vi "monte.fsk.vi"() -> ()   [LabVIEW 2014]
uses:
  <vilib>/Analysis/NI_AALBase.lvlib
panel:
  out "Waveform Chart":dbl(graph)
  in  "Numeric 4":i32
  in  "Numeric 2":i32
  out "BER":dbl format="%#_13g"
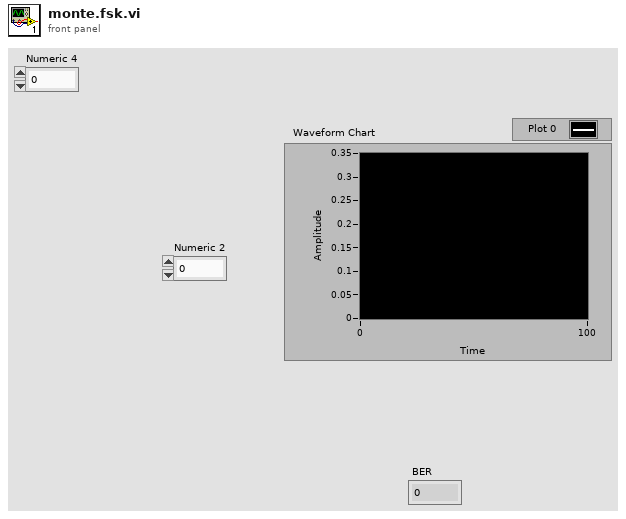
[diagram p1: front panel]
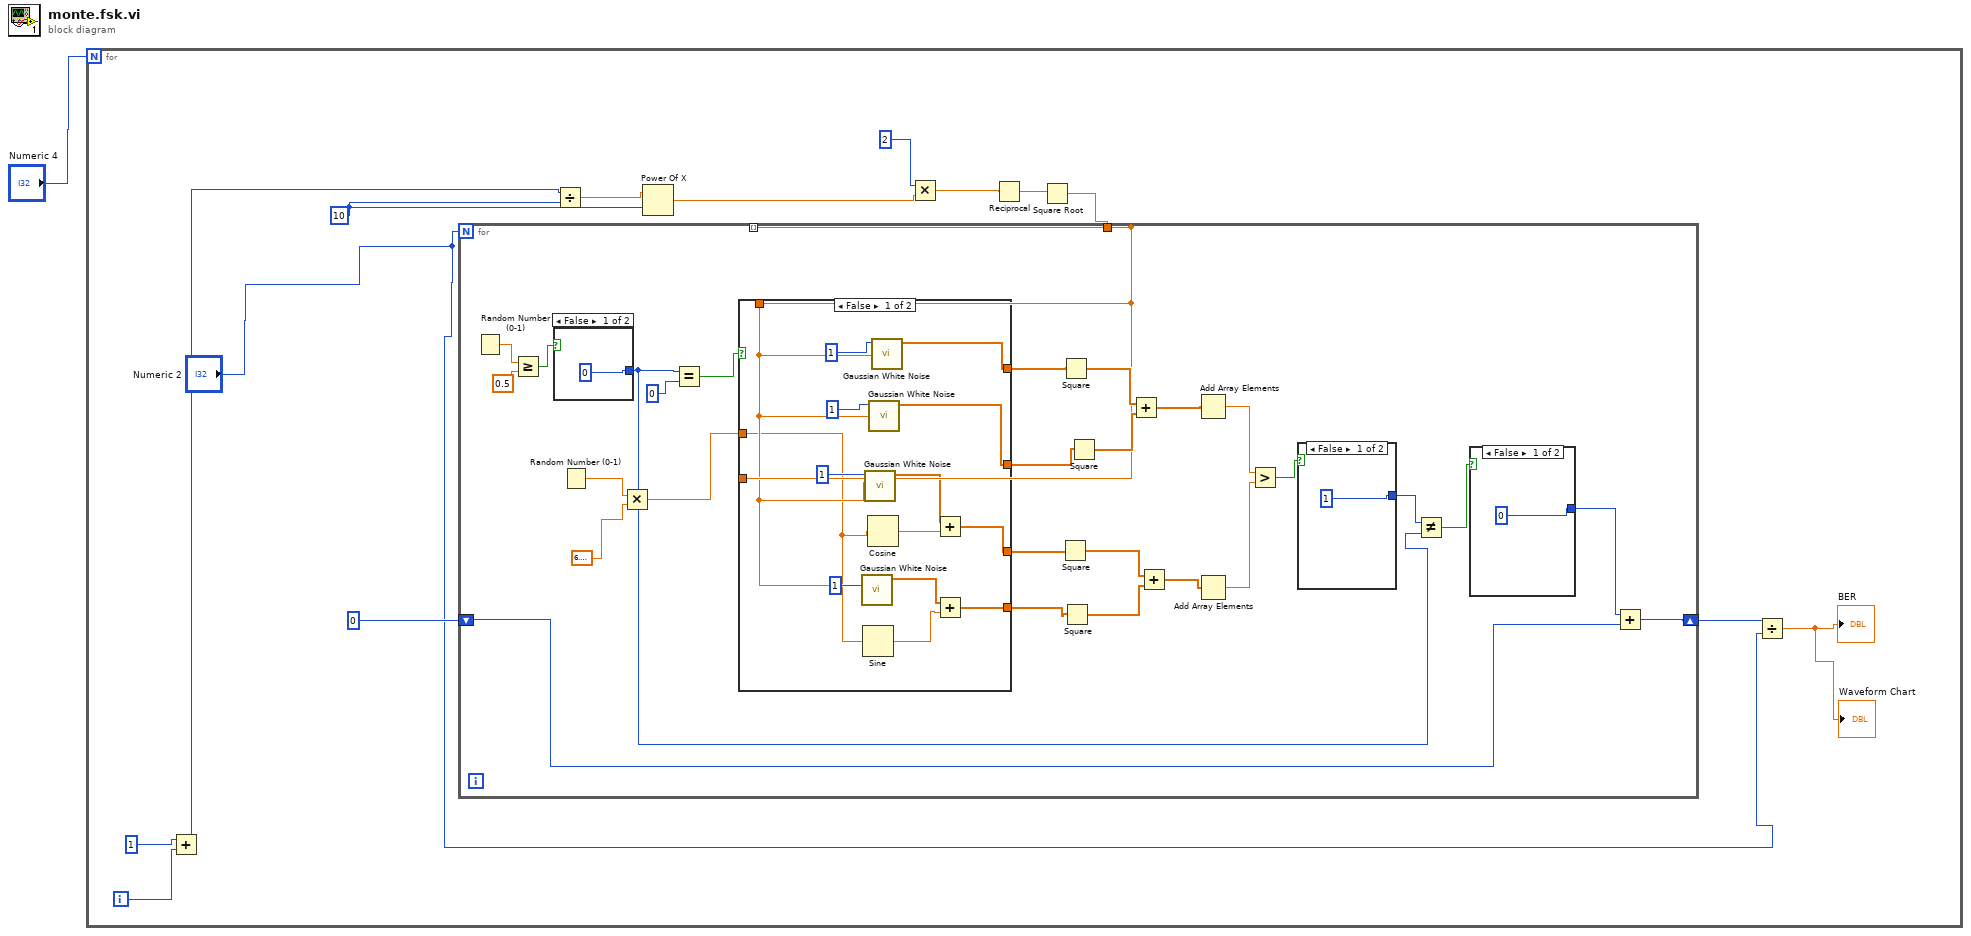
[diagram p0: block diagram]
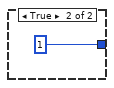
[diagram p2: hidden frame]
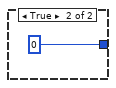
[diagram p3: hidden frame]
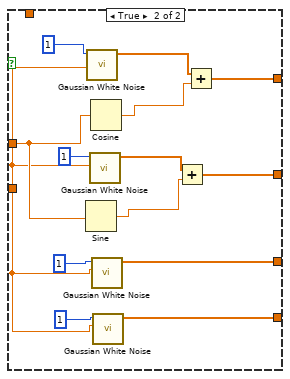
[diagram p4: hidden frame]
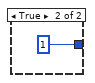
[diagram p5: hidden frame]
diagram:
  n1 = for {
    N: "Numeric 4" -> [_]
    i -> [w5]
    w13 = 10
    n2 = Add(x=1, y=w5) -> (x+y=w3:i32)
    n3 = Divide(x=w3, y=w13) -> (x/y=w14:dbl)
    n4 = Power Of X(1:w13, 2:w14) -> (0:w12:dbl)
    n5 = Multiply(x=2, y=w12) -> (x*y=w11:dbl)
    n6 = Reciprocal(x=w11) -> (1/x=w10:dbl)
    n7 = Square Root(x=w10) -> (sqrt(x)=w9:dbl)
    n8 = for {
      N: "Numeric 2" -> [_]
      shift-right: [w19] -> w15
      shift-left: 0 -> [w18]
      tunnel: [w16] -> _ mode=indexing
      tunnel: w9 -> [w16]
      n9 = Random Number (0-1)() -> (number: 0 to 1=w42:dbl)
      n10 = Greater Or Equal?(x=w42, y=0.5) -> (x >= y?=w43:bool)
      n11 = case shown="False" w43 {
        tunnel: [0 1] -> w21
        frame False {
        }
        frame True {
        }
      }
      n12 = Random Number (0-1)() -> (number: 0 to 1=w38:dbl)
      n13 = Multiply(x=w38, y=6.283185307179586) -> (x*y=w37:dbl)
      n14 = Equal?(x=w21, y=0) -> (x = y?=w39:bool)
      n15 = case shown="False" w39 {
        tunnel: w37 -> [w48 w63]
        tunnel: [w51 w74] -> w36
        tunnel: [w52 w71] -> w35
        tunnel: [w53 w70] -> w34
        tunnel: [w56 w69] -> w33
        tunnel: w16 -> [_ w62]
        tunnel: w16 -> [w49 _]
        frame False {
          n16 = call <vilib>:"Gaussian White Noise.vi"("standard deviation"=w49, "samples"=1) -> ("Gaussian noise pattern"=w58:dbl[])  [unwired: 8 in, 1 out]
          n17 = Sine(x=w48) -> (sin(x)=w57:dbl)
          n18 = call <vilib>:"Gaussian White Noise.vi"("standard deviation"=w49, "samples"=1) -> ("Gaussian noise pattern"=w54:dbl[])  [unwired: 8 in, 1 out]
          n19 = Cosine(x=w48) -> (cos(x)=w55:dbl)
          n20 = call <vilib>:"Gaussian White Noise.vi"("standard deviation"=w49, "samples"=1) -> ("Gaussian noise pattern"=w52:dbl[])  [unwired: 8 in, 1 out]
          n21 = call <vilib>:"Gaussian White Noise.vi"("standard deviation"=w49, "samples"=1) -> ("Gaussian noise pattern"=w51:dbl[])  [unwired: 8 in, 1 out]
          n22 = Add(x=w54, y=w55) -> (x+y=w53:dbl[])
          n23 = Add(x=w58, y=w57) -> (x+y=w56:dbl[])
        }
        frame True {
          n24 = Sine(x=w63) -> (sin(x)=w64:dbl)
          n25 = call <vilib>:"Gaussian White Noise.vi"("standard deviation"=w62, "samples"=1) -> ("Gaussian noise pattern"=w75:dbl[])  [unwired: 8 in, 1 out]
          n26 = call <vilib>:"Gaussian White Noise.vi"("standard deviation"=w62, "samples"=1) -> ("Gaussian noise pattern"=w72:dbl[])  [unwired: 8 in, 1 out]
          n27 = Cosine(x=w63) -> (cos(x)=w65:dbl)
          n28 = call <vilib>:"Gaussian White Noise.vi"("standard deviation"=w62, "samples"=1) -> ("Gaussian noise pattern"=w70:dbl[])  [unwired: 8 in, 1 out]
          n29 = call <vilib>:"Gaussian White Noise.vi"("standard deviation"=w62, "samples"=1) -> ("Gaussian noise pattern"=w69:dbl[])  [unwired: 8 in, 1 out]
          n30 = Add(x=w72, y=w64) -> (x+y=w71:dbl[])
          n31 = Add(x=w75, y=w65) -> (x+y=w74:dbl[])
        }
      }
      n32 = Square(x=w34) -> (x^2=w30:dbl[])
      n33 = Square(x=w36) -> (x^2=w32:dbl[])
      n34 = Square(x=w33) -> (x^2=w29:dbl[])
      n35 = Square(x=w35) -> (x^2=w31:dbl[])
      n36 = Add(x=w32, y=w31) -> (x+y=w28:dbl[])
      n37 = Add(x=w30, y=w29) -> (x+y=w27:dbl[])
      n38 = Add Array Elements(numeric array=w28) -> (sum=w26:dbl)
      n39 = Add Array Elements(numeric array=w27) -> (sum=w25:dbl)
      n40 = Greater?(x=w26, y=w25) -> (0:w24:bool)
      n41 = case shown="False" w24 {
        tunnel: [1 0] -> w22
        frame False {
        }
        frame True {
        }
      }
      n42 = Not Equal?(x=w22, y=w21) -> (x != y?=w23:bool)
      n43 = case shown="False" w23 {
        tunnel: [0 1] -> w20
        frame False {
        }
        frame True {
        }
      }
      n44 = Add(x=w20, y=w18) -> (x+y=w19:i32)
    }
    n45 = Divide(x=w15, y="Numeric 2") -> (x/y=→"BER" →"Waveform Chart":dbl)
  }
